vi "Dresden Edit Recipe(in).vi"() -> ()   [LabVIEW 2009] (continued)
              n2343 = Format Into String(format string="%s%s%s%s%.1f", "\r", "Maximum Diameter(mm):" ("input 2"), w2767, w2767, w2766) -> (resulting string=w2765:string)  [unwired: 2 in, 1 out]
            }
            frame #7 {
              w2773 = "\t"
              n2344 = local read "R Web thickness"() -> (w2772:dbl)
              n2345 = Format Into String(format string="%s%s%s%s%d", "\r", "Web Thickness(µm):" ("input 2"), w2773, w2773, w2772) -> (resulting string=w2771:string)  [unwired: 2 in, 1 out]
            }
            frame #8 {
              w2779 = "\t"
              n2346 = local read "R Web speed(cm/min)"() -> (w2778:dbl)
              n2347 = Format Into String(format string="%s%s%s%s%d", "\r", "Web Speed(cm/min):" ("input 2"), w2779, w2779, w2778) -> (resulting string=w2777:string)  [unwired: 2 in, 1 out]
            }
            frame #9 {
              w2785 = "\t"
              n2348 = local read "R Tension Value"() -> (w2784:dbl)
              n2349 = Format Into String(format string="%s%s%s%s%d", "\r", "Tension Value(N):" ("input 2"), w2785, w2785, w2784) -> (resulting string=w2783:string)  [unwired: 2 in, 1 out]
            }
            frame #10 {
              w2791 = "\r"
              w2792 = "\t"
              n2350 = local read "R  Total length"() -> (w2790:dbl)
              n2351 = Format Into String(format string="%s%s%s%s%s%.1f%s%s", "\r", "Total Length:" ("input 2"), w2792, w2792, w2792, w2790, w2791, w2791) -> (resulting string=w2789:string)  [unwired: 2 in, 1 out]
            }
            frame #11 {
              w2798 = "\t"
              n2352 = Format Into String(format string="%s%s%s%s", "Other Parameters" ("input 1"), w2798, w2798, "\r") -> (resulting string=w2796:string)  [unwired: 2 in, 1 out]
            }
            frame #12 {
              w2802 = "\t"
              n2353 = local read "R_Thickness Selection"() -> (w2806:enum32{"Thickness", "Time"})
              n2354 = case shown="\"Thickness\", Default" w2806 {
                tunnel: ["Thickness" ("input 3") "Time" ("input 3")] -> w2803
                frame #0 {
                }
                frame #1 {
                }
              }
              n2355 = Format Into String(format string="%s%s%s%s", "Thickness Selection:" ("input 1"), w2802, w2802, w2803) -> (resulting string=w2801:string)  [unwired: 2 in, 1 out]
            }
            frame #13 {
              n2356 = local read "R_Target Thickness Value"() -> (w2810:dbl)
              n2357 = Format Into String(format string="%s%s%s%d", "\r", "Target Thicness Value(nm):" ("input 2"), "\t", w2810) -> (resulting string=w2809:string)  [unwired: 2 in, 1 out]
            }
            frame #14 {
              w2816 = "\r"
              w2818 = "\t"
              n2358 = local read "R_Duration"() -> (w2817:dbl)
              n2359 = Format Into String(format string="%s%s%s%s%s%d%s%s", "\r", "Time(s):" ("input 2"), w2818, w2818, w2818, w2817, w2816, w2816) -> (resulting string=w2815:string)  [unwired: 2 in, 1 out]
            }
            frame #15 {
              w2824 = "\t"
              n2360 = Format Into String(format string="%s%s%s%s", "Single Recipe Parameters" ("input 1"), w2824, w2824, "\r") -> (resulting string=w2822:string)  [unwired: 2 in, 1 out]
            }
            frame #16 {
              n2361 = local read "R_Simple_Coating Type Selection"() -> (w2830:T2)
              n2362 = case shown="\"Microwave Plasma\", Default" w2830 {
                tunnel: ["Microwave Plasma" ("string") "DC Sputter" ("string") "RF Sputter" ("string")] -> w2828
                frame #0 {
                }
                frame #1 {
                }
                frame #2 {
                }
              }
              n2363 = Format Into String(format string="%s%s%s%s", "Single  Process Selection:" ("input 1"), "\t", w2828, "\r") -> (resulting string=w2829:string)  [unwired: 2 in, 1 out]
            }
            frame #17 {
              w2838 = "\t"
              n2364 = Format Into String(format string="%s%s%s", "Microwave Plasma Parameters" ("input 1"), w2838, w2838) -> (resulting string=w2837:string)  [unwired: 2 in, 1 out]
            }
            frame #18 {
              n2365 = local read "R_Single Microwave Power"() -> (w2842:dbl)
              n2366 = Format Into String(format string="%s%s%s%d", "\r", "Microwave Plasma Power(W):" ("input 2"), "\t", w2842) -> (resulting string=w2841:string)  [unwired: 2 in, 1 out]
            }
            frame #19 {
              n2367 = local read "R_Single Microwave Time"() -> (w2848:dbl)
              n2368 = Format Into String(format string="%s%s%s%d", "\r", "Microwave Plasma Time(s):" ("input 2"), "\t", w2848) -> (resulting string=w2847:string)  [unwired: 2 in, 1 out]
            }
            frame #20 {
              w2853 = "\r"
              w2856 = "\t"
              n2369 = local read "R Single Pass Number"() -> (w2854:dbl)
              n2370 = Format Into String(format string="%s%s%s%s%s%d%s%s", "\r", "Pass Number:" ("input 2"), w2856, w2856, w2856, w2854, w2853, w2853) -> (resulting string=w2855:string)  [unwired: 2 in, 1 out]
            }
            frame #21 {
              w2861 = "\r"
              w2862 = "\t"
              n2371 = Format Into String(format string="%s%s%s%s%s", "DC Sputter Parameters" ("input 1"), w2862, w2862, w2861, w2861) -> (resulting string=w2860:string)  [unwired: 2 in, 1 out]
            }
            frame #22 {
              w2869 = "\t"
              n2372 = local read "R_DC_Chamber_selection"() -> (w2867:enum32{"Chamber II", "Chamber III"})
              n2373 = case shown="\"Chamber II\", Default" w2867 {
                tunnel: ["Chamber II" ("string") "Chamber III" ("string")] -> w2868
                frame #0 {
                }
                frame #1 {
                }
              }
              n2374 = Format Into String(format string="%s%s%s%s%s%s", "\r", "DC Chamber Selection :" ("input 2"), w2869, w2869, w2868, "\r") -> (resulting string=w2865:string)  [unwired: 2 in, 1 out]
            }
            frame #23 {
              w2877 = "\t"
              n2375 = local read "R Single DC Target material"() -> (w2876:string)
              n2376 = Format Into String(format string="%s%s%s%s", "Target Material:" ("string"), w2877, w2877, w2876) -> (resulting string=w2875:string)  [unwired: 2 in, 1 out]
            }
            frame #24 {
              w2882 = "\t"
              n2377 = local read "R Single DC Step1 Coating Power Active"() -> (w2883:bool)
              n2378 = case shown="True" w2883 {
                tunnel: ["Deactive" ("input 4") "Active" ("input 4")] -> w2881
                frame #0 {
                }
                frame #1 {
                }
              }
              n2379 = Format Into String(format string="%s%s%s%s%s%s", "\r", "Region 1:" ("input 2"), w2882, w2882, w2882, w2881) -> (resulting string=w2880:string)  [unwired: 2 in, 1 out]
            }
            frame #25 {
              w2894 = "\t"
              n2380 = local read "R Single DC Step1 Coating Power"() -> (w2890:dbl)
              n2381 = Format Into String(format string="%s%s%s%s%s%d", "\r", "Power(W):" ("input 2"), w2894, w2894, w2894, w2890) -> (resulting string=w2889:string)  [unwired: 2 in, 1 out]
            }
            frame #26 {
              w2897 = "\t"
              n2382 = local read "R Single DC Interval length1"() -> (w2896:dbl)
              n2383 = Format Into String(format string="%s%s%s%s%d", "\r", "Interval Length(m):" ("input 2"), w2897, w2897, w2896) -> (resulting string=w2895:string)  [unwired: 2 in, 1 out]
            }
            frame #27 {
              w2902 = "\t"
              n2384 = local read "R Single DC Step2 Coating Power Active"() -> (w2904:bool)
              n2385 = case shown="True" w2904 {
                tunnel: ["Deactive" ("input 4") "Active" ("input 4")] -> w2903
                frame #0 {
                }
                frame #1 {
                }
              }
              n2386 = Format Into String(format string="%s%s%s%s%s%s", "\r", "Region 2:" ("input 2"), w2902, w2902, w2902, w2903) -> (resulting string=w2901:string)  [unwired: 2 in, 1 out]
            }
            frame #28 {
              w2915 = "\t"
              n2387 = local read "R Single DC Step2 Coating Power"() -> (w2911:dbl)
              n2388 = Format Into String(format string="%s%s%s%s%s%d", "\r", "Power(W):" ("input 2"), w2915, w2915, w2915, w2911) -> (resulting string=w2910:string)  [unwired: 2 in, 1 out]
            }
            frame #29 {
              w2918 = "\t"
              n2389 = local read "R Single DC Interval length2"() -> (w2917:dbl)
              n2390 = Format Into String(format string="%s%s%s%s%d", "\r", "Interval Length(m):" ("input 2"), w2918, w2918, w2917) -> (resulting string=w2916:string)  [unwired: 2 in, 1 out]
            }
            frame #30 {
              w2924 = "\t"
              n2391 = local read "R Single DC Step3 Coating Power Active"() -> (w2925:bool)
              n2392 = case shown="True" w2925 {
                tunnel: ["Deactive" ("input 4") "Active" ("input 4")] -> w2923
                frame #0 {
                }
                frame #1 {
                }
              }
              n2393 = Format Into String(format string="%s%s%s%s%s%s", "\r", "Region 3:" ("input 2"), w2924, w2924, w2924, w2923) -> (resulting string=w2922:string)  [unwired: 2 in, 1 out]
            }
            frame #31 {
              w2936 = "\t"
              n2394 = local read "R Single DC Step3 Coating Power"() -> (w2931:dbl)
              n2395 = Format Into String(format string="%s%s%s%s%s%d", "\r", "Power(W):" ("input 2"), w2936, w2936, w2936, w2931) -> (resulting string=w2932:string)  [unwired: 2 in, 1 out]
            }
            frame #32 {
              w2939 = "\t"
              n2396 = local read "R Single DC Interval length3"() -> (w2938:dbl)
              n2397 = Format Into String(format string="%s%s%s%s%d", "\r", "Interval Length(m):" ("input 2"), w2939, w2939, w2938) -> (resulting string=w2937:string)  [unwired: 2 in, 1 out]
            }
            frame #33 {
              w2944 = "\t"
              n2398 = local read "R Single DC Step4 Coating Power Active"() -> (w2946:bool)
              n2399 = case shown="True" w2946 {
                tunnel: ["Deactive" ("input 4") "Active" ("input 4")] -> w2945
                frame #0 {
                }
                frame #1 {
                }
              }
              n2400 = Format Into String(format string="%s%s%s%s%s%s", "\r", "Region 4:" ("input 2"), w2944, w2944, w2944, w2945) -> (resulting string=w2943:string)  [unwired: 2 in, 1 out]
            }
            frame #34 {
              w2957 = "\t"
              n2401 = local read "R Single DC Step4 Coating Power"() -> (w2952:dbl)
              n2402 = Format Into String(format string="%s%s%s%s%s%d", "\r", "Power(W):" ("input 2"), w2957, w2957, w2957, w2952) -> (resulting string=w2953:string)  [unwired: 2 in, 1 out]
            }
            frame #35 {
              w2960 = "\t"
              n2403 = local read "R Single DC Interval length4"() -> (w2959:dbl)
              n2404 = Format Into String(format string="%s%s%s%s%d", "\r", "Interval Length(m):" ("input 2"), w2960, w2960, w2959) -> (resulting string=w2958:string)  [unwired: 2 in, 1 out]
            }
            frame #36 {
              w2965 = "\t"
              n2405 = local read "R Single DC Step5 Coating Power Active"() -> (w2967:bool)
              n2406 = case shown="True" w2967 {
                tunnel: ["Deactive" ("input 4") "Active" ("input 4")] -> w2966
                frame #0 {
                }
                frame #1 {
                }
              }
              n2407 = Format Into String(format string="%s%s%s%s%s%s", "\r", "Region 5:" ("input 2"), w2965, w2965, w2965, w2966) -> (resulting string=w2964:string)  [unwired: 2 in, 1 out]
            }
            frame #37 {
              w2978 = "\t"
              n2408 = local read "R Single DC Step5 Coating Power"() -> (w2973:dbl)
              n2409 = Format Into String(format string="%s%s%s%s%s%d", "\r", "Power(W):" ("input 2"), w2978, w2978, w2978, w2973) -> (resulting string=w2974:string)  [unwired: 2 in, 1 out]
            }
            frame #38 {
              w2981 = "\t"
              n2410 = local read "R Single DC Interval length5"() -> (w2980:dbl)
              n2411 = Format Into String(format string="%s%s%s%s%d", "\r", "Interval Length(m):" ("input 2"), w2981, w2981, w2980) -> (resulting string=w2979:string)  [unwired: 2 in, 1 out]
            }
            frame #39 {
              w2986 = "\t"
              n2412 = local read "R Single DC Step6 Coating Power Active"() -> (w2988:bool)
              n2413 = case shown="True" w2988 {
                tunnel: ["Deactive" ("input 4") "Active" ("input 4")] -> w2987
                frame #0 {
                }
                frame #1 {
                }
              }
              n2414 = Format Into String(format string="%s%s%s%s%s%s", "\r", "Region 6:" ("input 2"), w2986, w2986, w2986, w2987) -> (resulting string=w2985:string)  [unwired: 2 in, 1 out]
            }
            frame #40 {
              w2999 = "\t"
              n2415 = local read "R Single DC Step6 Coating Power"() -> (w2994:dbl)
              n2416 = Format Into String(format string="%s%s%s%s%s%d", "\r", "Power(W):" ("input 2"), w2999, w2999, w2999, w2994) -> (resulting string=w2995:string)  [unwired: 2 in, 1 out]
            }
            frame #41 {
              w3002 = "\t"
              n2417 = local read "R Single DC Interval length6"() -> (w3001:dbl)
              n2418 = Format Into String(format string="%s%s%s%s%d", "\r", "Interval Length(m):" ("input 2"), w3002, w3002, w3001) -> (resulting string=w3000:string)  [unwired: 2 in, 1 out]
            }
            frame #42 {
              w3007 = "\t"
              n2419 = local read "R Single DC Step7 Coating Power Active"() -> (w3009:bool)
              n2420 = case shown="True" w3009 {
                tunnel: ["Deactive" ("input 4") "Active" ("input 4")] -> w3008
                frame #0 {
                }
                frame #1 {
                }
              }
              n2421 = Format Into String(format string="%s%s%s%s%s%s", "\r", "Region 7:" ("input 2"), w3007, w3007, w3007, w3008) -> (resulting string=w3006:string)  [unwired: 2 in, 1 out]
            }
            frame #43 {
              w3020 = "\t"
              n2422 = local read "R Single DC Step7 Coating Power"() -> (w3015:dbl)
              n2423 = Format Into String(format string="%s%s%s%s%s%d", "\r", "Power(W):" ("input 2"), w3020, w3020, w3020, w3015) -> (resulting string=w3016:string)  [unwired: 2 in, 1 out]
            }
            frame #44 {
              w3023 = "\t"
              n2424 = local read "R Single DC Interval length7"() -> (w3022:dbl)
              n2425 = Format Into String(format string="%s%s%s%s%d", "\r", "Interval Length(m):" ("input 2"), w3023, w3023, w3022) -> (resulting string=w3021:string)  [unwired: 2 in, 1 out]
            }
            frame #45 {
              w3028 = "\t"
              n2426 = local read "R Single DC Step8 Coating Power Active"() -> (w3030:bool)
              n2427 = case shown="True" w3030 {
                tunnel: ["Deactive" ("input 4") "Active" ("input 4")] -> w3029
                frame #0 {
                }
                frame #1 {
                }
              }
              n2428 = Format Into String(format string="%s%s%s%s%s%s", "\r", "Region 8:" ("input 2"), w3028, w3028, w3028, w3029) -> (resulting string=w3027:string)  [unwired: 2 in, 1 out]
            }
            frame #46 {
              w3041 = "\t"
              n2429 = local read "R Single DC Step8 Coating Power"() -> (w3036:dbl)
              n2430 = Format Into String(format string="%s%s%s%s%s%d", "\r", "Power(W):" ("input 2"), w3041, w3041, w3041, w3036) -> (resulting string=w3037:string)  [unwired: 2 in, 1 out]
            }
            frame #47 {
              w3044 = "\t"
              n2431 = local read "R Single DC Interval length8"() -> (w3043:dbl)
              n2432 = Format Into String(format string="%s%s%s%s%d", "\r", "Interval Length(m):" ("input 2"), w3044, w3044, w3043) -> (resulting string=w3042:string)  [unwired: 2 in, 1 out]
            }
            frame #48 {
              w3049 = "\t"
              n2433 = local read "R Single DC Step9 Coating Power Active"() -> (w3051:bool)
              n2434 = case shown="True" w3051 {
                tunnel: ["Deactive" ("input 4") "Active" ("input 4")] -> w3050
                frame #0 {
                }
                frame #1 {
                }
              }
              n2435 = Format Into String(format string="%s%s%s%s%s%s", "\r", "Region 9:" ("input 2"), w3049, w3049, w3049, w3050) -> (resulting string=w3048:string)  [unwired: 2 in, 1 out]
            }
            frame #49 {
              w3062 = "\t"
              n2436 = local read "R Single DC Step9 Coating Power"() -> (w3058:dbl)
              n2437 = Format Into String(format string="%s%s%s%s%s%d", "\r", "Power(W):" ("input 2"), w3062, w3062, w3062, w3058) -> (resulting string=w3057:string)  [unwired: 2 in, 1 out]
            }
            frame #50 {
              w3065 = "\t"
              n2438 = local read "R Single DC Interval length9"() -> (w3064:dbl)
              n2439 = Format Into String(format string="%s%s%s%s%d", "\r", "Interval Length(m):" ("input 2"), w3065, w3065, w3064) -> (resulting string=w3063:string)  [unwired: 2 in, 1 out]
            }
            frame #51 {
              w3070 = "\t"
              n2440 = local read "R Single DC Step10 Coating Power Active"() -> (w3072:bool)
              n2441 = case shown="True" w3072 {
                tunnel: ["Deactive" ("input 4") "Active" ("input 4")] -> w3071
                frame #0 {
                }
                frame #1 {
                }
              }
              n2442 = Format Into String(format string="%s%s%s%s%s%s", "\r", "Region 10:" ("input 2"), w3070, w3070, w3070, w3071) -> (resulting string=w3069:string)  [unwired: 2 in, 1 out]
            }
            frame #52 {
              w3083 = "\t"
              n2443 = local read "R Single DC Step10 Coating Power"() -> (w3078:dbl)
              n2444 = Format Into String(format string="%s%s%s%s%s%d", "\r", "Power(W):" ("input 2"), w3083, w3083, w3083, w3078) -> (resulting string=w3079:string)  [unwired: 2 in, 1 out]
            }
            frame #53 {
              w3085 = "\r"
              w3087 = "\t"
              n2445 = local read "R Single DC Interval length10"() -> (w3086:dbl)
              n2446 = Format Into String(format string="%s%s%s%s%d%s%s", "\r", "Interval Length(m):" ("input 2"), w3087, w3087, w3086, w3085, w3085) -> (resulting string=w3084:string)  [unwired: 2 in, 1 out]
            }
            frame #54 {
              w3092 = "\t"
              n2447 = Format Into String(format string="%s%s%s", "RF Sputter Parameters" ("input 1"), w3092, w3092) -> (resulting string=w3091:string)  [unwired: 2 in, 1 out]
            }
            frame #55 {
              w3097 = "\t"
              n2448 = local read "R Single RF Target material"() -> (w3096:string)
              n2449 = Format Into String(format string="%s%s%s%s%s", "\r", "Target Material:" ("input 2"), w3097, w3097, w3096) -> (resulting string=w3095:string)  [unwired: 2 in, 1 out]
            }
            frame #56 {
              w3104 = "\t"
              n2450 = local read "R Single RF Ramp up"() -> (w3102:bool)
              n2451 = case shown="True" w3102 {
                tunnel: ["Deactive" ("input 4") "Active" ("input 4")] -> w3103
                frame #0 {
                }
                frame #1 {
                }
              }
              n2452 = Format Into String(format string="%s%s%s%s%s", "\r", "Ramp Up Time(s):" ("input 2"), w3104, w3104, w3103) -> (resulting string=w3101:string)  [unwired: 2 in, 1 out]
            }
            frame #57 {
              w3112 = "\t"
              n2453 = local read "R Single RF Ramp up Time"() -> (w3111:dbl)
              n2454 = Format Into String(format string="%s%s%s%s%d", "\r", "Ramp Up Time(s):" ("input 2"), w3112, w3112, w3111) -> (resulting string=w3110:string)  [unwired: 2 in, 1 out]
            }
            frame #58 {
              w3117 = "\t"
              n2455 = local read "R Single RF Step1 Coating Power Active"() -> (w3119:bool)
              n2456 = case shown="False" w3119 {
                tunnel: ["Deactive" ("input 4") "Active" ("input 4")] -> w3118
                frame #0 {
                }
                frame #1 {
                }
              }
              n2457 = Format Into String(format string="%s%s%s%s%s%s", "\r", "Region 1:" ("input 2"), w3117, w3117, w3117, w3118) -> (resulting string=w3116:string)  [unwired: 2 in, 1 out]
            }
            frame #59 {
              w3130 = "\t"
              n2458 = local read "R Single RF  Step1 Coating Power"() -> (w3126:dbl)
              n2459 = Format Into String(format string="%s%s%s%s%s%d", "\r", "Power(W):" ("input 2"), w3130, w3130, w3130, w3126) -> (resulting string=w3125:string)  [unwired: 2 in, 1 out]
            }
            frame #60 {
              w3133 = "\t"
              n2460 = local read "R Single RF Interval length"() -> (w3132:dbl)
              n2461 = Format Into String(format string="%s%s%s%s%d", "\r", "Interval Length(m):" ("input 2"), w3133, w3133, w3132) -> (resulting string=w3131:string)  [unwired: 2 in, 1 out]
            }
            frame #61 {
              w3138 = "\t"
              n2462 = local read "R Single RF Step2 Coating Power Active"() -> (w3140:bool)
              n2463 = case shown="False" w3140 {
                tunnel: ["Deactive" ("input 4") "Active" ("input 4")] -> w3139
                frame #0 {
                }
                frame #1 {
                }
              }
              n2464 = Format Into String(format string="%s%s%s%s%s%s", "\r", "Region 2:" ("input 2"), w3138, w3138, w3138, w3139) -> (resulting string=w3137:string)  [unwired: 2 in, 1 out]
            }
            frame #62 {
              w3151 = "\t"
              n2465 = local read "R Single RF Step2 Coating Power"() -> (w3146:dbl)
              n2466 = Format Into String(format string="%s%s%s%s%s%d", "\r", "Power(W):" ("input 2"), w3151, w3151, w3151, w3146) -> (resulting string=w3147:string)  [unwired: 2 in, 1 out]
            }
            frame #63 {
              w3154 = "\t"
              n2467 = local read "R Single RF Interval length2"() -> (w3153:dbl)
              n2468 = Format Into String(format string="%s%s%s%s%d", "\r", "Interval Length(m):" ("input 2"), w3154, w3154, w3153) -> (resulting string=w3152:string)  [unwired: 2 in, 1 out]
            }
            frame #64 {
              w3159 = "\t"
              n2469 = local read "R Single RF Step3 Coating Power Active"() -> (w3161:bool)
              n2470 = case shown="False" w3161 {
                tunnel: ["Deactive" ("input 4") "Active" ("input 4")] -> w3160
                frame #0 {
                }
                frame #1 {
                }
              }
              n2471 = Format Into String(format string="%s%s%s%s%s%s", "\r", "Region 3:" ("input 2"), w3159, w3159, w3159, w3160) -> (resulting string=w3158:string)  [unwired: 2 in, 1 out]
            }
            frame #65 {
              w3172 = "\t"
              n2472 = local read "R Single RF Step3 Coating Power"() -> (w3167:dbl)
              n2473 = Format Into String(format string="%s%s%s%s%s%d", "\r", "Power(W):" ("input 2"), w3172, w3172, w3172, w3167) -> (resulting string=w3168:string)  [unwired: 2 in, 1 out]
            }
            frame #66 {
              w3175 = "\t"
              n2474 = local read "R Single RF Interval length3"() -> (w3174:dbl)
              n2475 = Format Into String(format string="%s%s%s%s%d", "\r", "Interval Length(m):" ("input 2"), w3175, w3175, w3174) -> (resulting string=w3173:string)  [unwired: 2 in, 1 out]
            }
            frame #67 {
              w3180 = "\t"
              n2476 = local read "R Single RF Step4 Coating Power Active"() -> (w3182:bool)
              n2477 = case shown="False" w3182 {
                tunnel: ["Deactive" ("input 4") "Active" ("input 4")] -> w3181
                frame #0 {
                }
                frame #1 {
                }
              }
              n2478 = Format Into String(format string="%s%s%s%s%s%s", "\r", "Region 4:" ("input 2"), w3180, w3180, w3180, w3181) -> (resulting string=w3179:string)  [unwired: 2 in, 1 out]
            }
            frame #68 {
              w3193 = "\t"
              n2479 = local read "R Single RF Step4 Coating Power"() -> (w3188:dbl)
              n2480 = Format Into String(format string="%s%s%s%s%s%d", "\r", "Power(W):" ("input 2"), w3193, w3193, w3193, w3188) -> (resulting string=w3189:string)  [unwired: 2 in, 1 out]
            }
            frame #69 {
              w3196 = "\t"
              n2481 = local read "R Single RF Interval length4"() -> (w3195:dbl)
              n2482 = Format Into String(format string="%s%s%s%s%d", "\r", "Interval Length(m):" ("input 2"), w3196, w3196, w3195) -> (resulting string=w3194:string)  [unwired: 2 in, 1 out]
            }
            frame #70 {
              w3202 = "\t"
              n2483 = local read "R Single RF Step5 Coating Power Active"() -> (w3203:bool)
              n2484 = case shown="False" w3203 {
                tunnel: ["Deactive" ("input 4") "Active" ("input 4")] -> w3201
                frame #0 {
                }
                frame #1 {
                }
              }
              n2485 = Format Into String(format string="%s%s%s%s%s%s", "\r", "Region 5:" ("input 2"), w3202, w3202, w3202, w3201) -> (resulting string=w3200:string)  [unwired: 2 in, 1 out]
            }
            frame #71 {
              w3214 = "\t"
              n2486 = local read "R Single RF Step5 Coating Power"() -> (w3209:dbl)
              n2487 = Format Into String(format string="%s%s%s%s%s%d", "\r", "Power(W):" ("input 2"), w3214, w3214, w3214, w3209) -> (resulting string=w3210:string)  [unwired: 2 in, 1 out]
            }
            frame #72 {
              w3217 = "\t"
              n2488 = local read "R Single RF Interval length5"() -> (w3216:dbl)
              n2489 = Format Into String(format string="%s%s%s%s%d", "\r", "Interval Length(m):" ("input 2"), w3217, w3217, w3216) -> (resulting string=w3215:string)  [unwired: 2 in, 1 out]
            }
            frame #73 {
              w3223 = "\t"
              n2490 = local read "R Single RF Step6 Coating Power Active"() -> (w3224:bool)
              n2491 = case shown="False" w3224 {
                tunnel: ["Deactive" ("input 4") "Active" ("input 4")] -> w3222
                frame #0 {
                }
                frame #1 {
                }
              }
              n2492 = Format Into String(format string="%s%s%s%s%s%s", "\r", "Region 6:" ("input 2"), w3223, w3223, w3223, w3222) -> (resulting string=w3221:string)  [unwired: 2 in, 1 out]
            }
            frame #74 {
              w3235 = "\t"
              n2493 = local read "R Single RF Step6 Coating Power"() -> (w3230:dbl)
              n2494 = Format Into String(format string="%s%s%s%s%s%d", "\r", "Power(W):" ("input 2"), w3235, w3235, w3235, w3230) -> (resulting string=w3231:string)  [unwired: 2 in, 1 out]
            }
            frame #75 {
              w3238 = "\t"
              n2495 = local read "R Single RF Interval length6"() -> (w3237:dbl)
              n2496 = Format Into String(format string="%s%s%s%s%d", "\r", "Interval Length(m):" ("input 2"), w3238, w3238, w3237) -> (resulting string=w3236:string)  [unwired: 2 in, 1 out]
            }
            frame #76 {
              w3244 = "\t"
              n2497 = local read "R Single RF Step7 Coating Power Active"() -> (w3245:bool)
              n2498 = case shown="False" w3245 {
                tunnel: ["Deactive" ("input 4") "Active" ("input 4")] -> w3243
                frame #0 {
                }
                frame #1 {
                }
              }
              n2499 = Format Into String(format string="%s%s%s%s%s%s", "\r", "Region 7:" ("input 2"), w3244, w3244, w3244, w3243) -> (resulting string=w3242:string)  [unwired: 2 in, 1 out]
            }
            frame #77 {
              w3256 = "\t"
              n2500 = local read "R Single RF Step7 Coating Power"() -> (w3251:dbl)
              n2501 = Format Into String(format string="%s%s%s%s%s%d", "\r", "Power(W):" ("input 2"), w3256, w3256, w3256, w3251) -> (resulting string=w3252:string)  [unwired: 2 in, 1 out]
            }
            frame #78 {
              w3259 = "\t"
              n2502 = local read "R Single RF Interval length7"() -> (w3258:dbl)
              n2503 = Format Into String(format string="%s%s%s%s%d", "\r", "Interval Length(m):" ("input 2"), w3259, w3259, w3258) -> (resulting string=w3257:string)  [unwired: 2 in, 1 out]
            }
            frame #79 {
              w3265 = "\t"
              n2504 = local read "R Single RF Step8 Coating Power Active"() -> (w3266:bool)
              n2505 = case shown="False" w3266 {
                tunnel: ["Deactive" ("input 4") "Active" ("input 4")] -> w3264
                frame #0 {
                }
                frame #1 {
                }
              }
              n2506 = Format Into String(format string="%s%s%s%s%s%s", "\r", "Region 8:" ("input 2"), w3265, w3265, w3265, w3264) -> (resulting string=w3263:string)  [unwired: 2 in, 1 out]
            }
            frame #80 {
              w3277 = "\t"
              n2507 = local read "R Single RF Step8 Coating Power"() -> (w3272:dbl)
              n2508 = Format Into String(format string="%s%s%s%s%s%d", "\r", "Power(W):" ("input 2"), w3277, w3277, w3277, w3272) -> (resulting string=w3273:string)  [unwired: 2 in, 1 out]
            }
            frame #81 {
              w3280 = "\t"
              n2509 = local read "R Single RF Interval length8"() -> (w3279:dbl)
              n2510 = Format Into String(format string="%s%s%s%s%d", "\r", "Interval Length(m):" ("input 2"), w3280, w3280, w3279) -> (resulting string=w3278:string)  [unwired: 2 in, 1 out]
            }
            frame #82 {
              w3286 = "\t"
              n2511 = local read "R Single RF Step9 Coating Power Active"() -> (w3287:bool)
              n2512 = case shown="False" w3287 {
                tunnel: ["Deactive" ("input 4") "Active" ("input 4")] -> w3285
                frame #0 {
                }
                frame #1 {
                }
              }
              n2513 = Format Into String(format string="%s%s%s%s%s%s", "\r", "Region 9:" ("input 2"), w3286, w3286, w3286, w3285) -> (resulting string=w3284:string)  [unwired: 2 in, 1 out]
            }
            frame #83 {
              w3298 = "\t"
              n2514 = local read "R Single RF Step9 Coating Power"() -> (w3293:dbl)
              n2515 = Format Into String(format string="%s%s%s%s%s%d", "\r", "Power(W):" ("input 2"), w3298, w3298, w3298, w3293) -> (resulting string=w3294:string)  [unwired: 2 in, 1 out]
            }
            frame #84 {
              w3301 = "\t"
              n2516 = local read "R Single RF Interval length9"() -> (w3300:dbl)
              n2517 = Format Into String(format string="%s%s%s%s%d", "\r", "Interval Length(m):" ("input 2"), w3301, w3301, w3300) -> (resulting string=w3299:string)  [unwired: 2 in, 1 out]
            }
            frame #85 {
              w3307 = "\t"
              n2518 = local read "R Single RF Step10 Coating Power Active"() -> (w3308:bool)
              n2519 = case shown="False" w3308 {
                tunnel: ["Deactive" ("input 4") "Active" ("input 4")] -> w3306
                frame #0 {
                }
                frame #1 {
                }
              }
              n2520 = Format Into String(format string="%s%s%s%s%s%s", "\r", "Region 10:" ("input 2"), w3307, w3307, w3307, w3306) -> (resulting string=w3305:string)  [unwired: 2 in, 1 out]
            }
            frame #86 {
              w3319 = "\t"
              n2521 = local read "R Single RF Step10 Coating Power"() -> (w3314:dbl)
              n2522 = Format Into String(format string="%s%s%s%s%s%d", "\r", "Power(W):" ("input 2"), w3319, w3319, w3319, w3314) -> (resulting string=w3315:string)  [unwired: 2 in, 1 out]
            }
            frame #87 {
              w3322 = "\t"
              n2523 = local read "R Single RF Interval length10"() -> (w3321:dbl)
              n2524 = Format Into String(format string="%s%s%s%s%d", "\r", "Interval Length(m):" ("input 2"), w3322, w3322, w3321) -> (resulting string=w3320:string)  [unwired: 2 in, 1 out]
            }
            frame #88 {
              w3329 = "\t"
              n2525 = local read "R Single RF Ramp down"() -> (w3328:bool)
              n2526 = case shown="False" w3328 {
                tunnel: ["Deactive" ("input 4") "Active" ("input 4")] -> w3327
                frame #0 {
